vi "get_if travel error.vi"(8 "error in (no error)":errorcluster, 11 "HGF_Agent.lvclass in":refnum<class "MoAgSy_AgentBase.lvclass">) -> (0 "error out":errorcluster, 2 "if travel error":T1(ring), 3 "HGF_Agent.lvclass out":refnum<class "MoAgSy_AgentBase.lvclass">)   [LabVIEW 2009, in "MoAgSy_Base.lvlib" / "MoAgSy_AgentBase.lvclass"]
uses:
  MoAgSy_AgentBase.lvclass
  MoAgSy_AgentBase.lvclass/MoAgSy_AgentBase.ctl
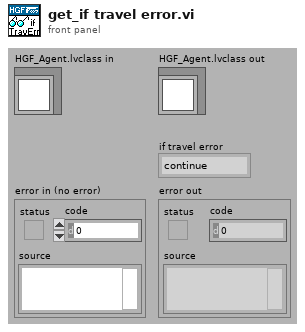
[diagram p1: front panel]
types:
  T1 = enum16{"continue", "shutdown", "nextDestination"}
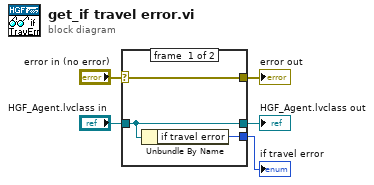
[diagram p0: block diagram]
diagram:
  n1 = case shown="No Error" "error in (no error)" {
    selector: "error in (no error)" -> [w8 w9]
    tunnel: [w8 w9] -> w4
    tunnel: [w7 w10] -> w2
    tunnel: "HGF_Agent.lvclass in" -> [w7 w10]
    tunnel: [w6 _] -> w1
    frame #0 {
      n2 = Unbundle By Name(w7) -> ("if travel error"=w6:T1)
    }
    frame #1 {
    }
  }
  "error out" <- w4
  "HGF_Agent.lvclass out" <- w2
  "if travel error" <- w1
